vi "AlazarSetParameterUL.vi"(0 "Handle":u32, 5 "Channel":u8(ring)=1 items=["A"=1, "B"=2, "C"=4, "D"=8], 7 "Parameter":u32(ring)=268435465 items=["Set ADC Mode"=268435527, "Data Width"=268435465, "Set/Get Async BuffSize"=268435513, "Set/Get Async Buffcount"=268435520, "Get Data Format"=268435522, "Get Samples Per Timestamp Clock"=268435524, "Get Records Captured"=268435525, "Get Async Buffers Pending"=268435536, "Get Async Buffers Pending Full"=268435537, "Get Async Buffers Pending Empty"=268435538, "ECC Mode"=268435528, "Get Aux Input Level"=268435529, "Get Channels Per Board"=268435568, "Pack Mode"=268435570, "Get FPGA Temperature"=268435584], 9 "Value":u32, 11 "error in (no error)":errorcluster) -> (4 "Handle":u32, 10 "Return Code":u32, 15 "error out":errorcluster)   [LabVIEW 2021]
doc: "Set a device parameter as an unsigned 32-bit value."
uses:
  ATSApi.dll
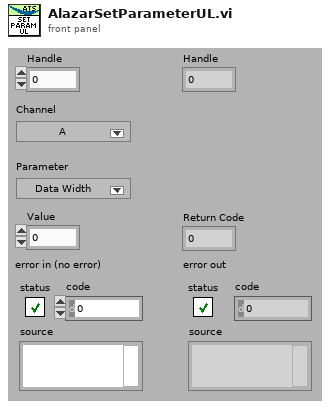
[diagram p1: front panel]
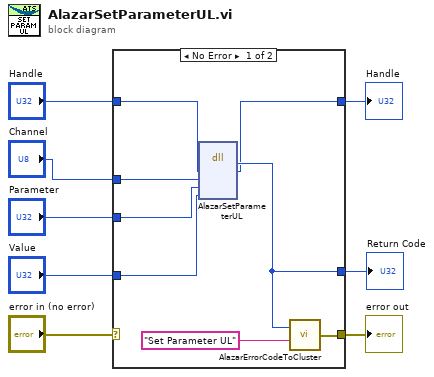
[diagram p0: block diagram]
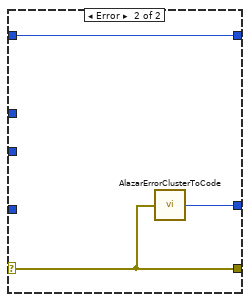
[diagram p2: hidden frame]
diagram:
  n1 = case shown="No Error" "error in (no error)" {
    selector: "error in (no error)" -> [_ w19]
    tunnel: [w13 w19] -> w7
    tunnel: [w15 w18] -> w6
    tunnel: "Handle" -> [w16 w17]
    tunnel: [w12 w17] -> w4
    tunnel: "Channel" -> [w11 _]
    tunnel: "Parameter" -> [w10 _]
    tunnel: "Value" -> [w9 _]
    frame No Error {
      n2 = dll-call lib="ATSApi.dll" fn="AlazarSetParameterUL"("handle"=w16, "channel"=w11, "parameter"=w10, "value"=w9) -> (w15:u32, "handle"=w12:u32)  [unwired: 6 in, 2 out]
      n3 = call "AlazarErrorCodeToCluster.vi"("Message"="Set Parameter UL", "Error Code"=w15) -> ("error out"=w13:errorcluster)
    }
    frame Error {
      n4 = call "AlazarErrorClusterToCode.vi"("error in (no error)"=w19) -> ("Error Code"=w18:u32)
    }
  }
  "Handle" <- w4
  "error out" <- w7
  "Return Code" <- w6
